vi "Unflatten Integer.vi"(11 "Tag value":string) -> (3 "Numeric":i32)   [LabVIEW 2020, in "NI_VIAn_XML Parsing.lvlib"]
uses:
  <vilib>/addons/analyzer/XML Parsing/NI_VIAn_XML Parsing.lvlib
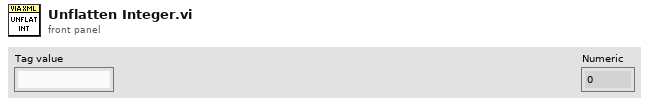
[diagram p1: front panel]
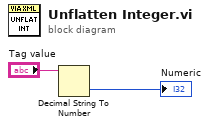
[diagram p0: block diagram]
diagram:
  n1 = Decimal String To Number(string="Tag value") -> (number=→"Numeric":i32)  [unwired: 2 in, 1 out]
